vi "examen.vi"() -> ()   [LabVIEW 2020]
uses:
  <vilib>/numeric/Random Number (Range) DBL.vi
panel:
  in  "?":dbl
  in  "LIMITE MINIMO":dbl
  in  "LIMITE MAXIMO":dbl
  out "VALOR HISTERESIS":bool
  out "señal":dynamicdata(graph)
  out "?":dbl
  out "VALOR":bool
  out "señal sin filtro":dbl
  in  "?":bool
  # "EXAMEN INSTRUMENTACION VIRTUAL"
  # "Max."
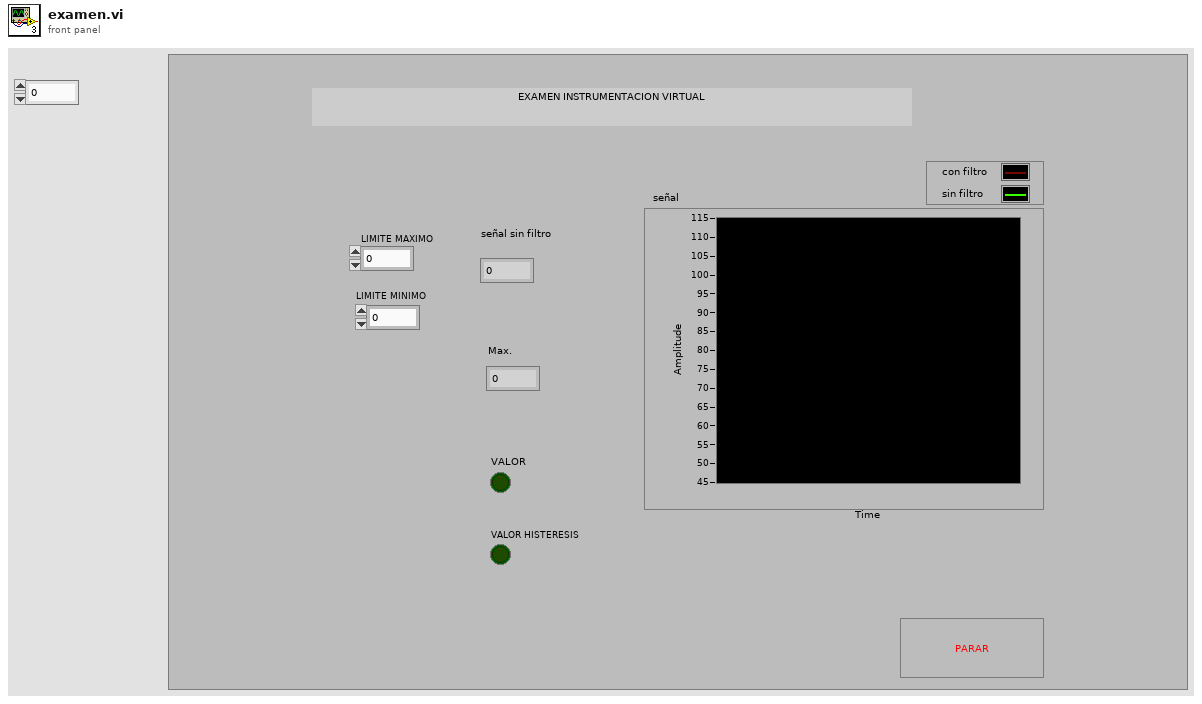
[diagram p1: front panel]
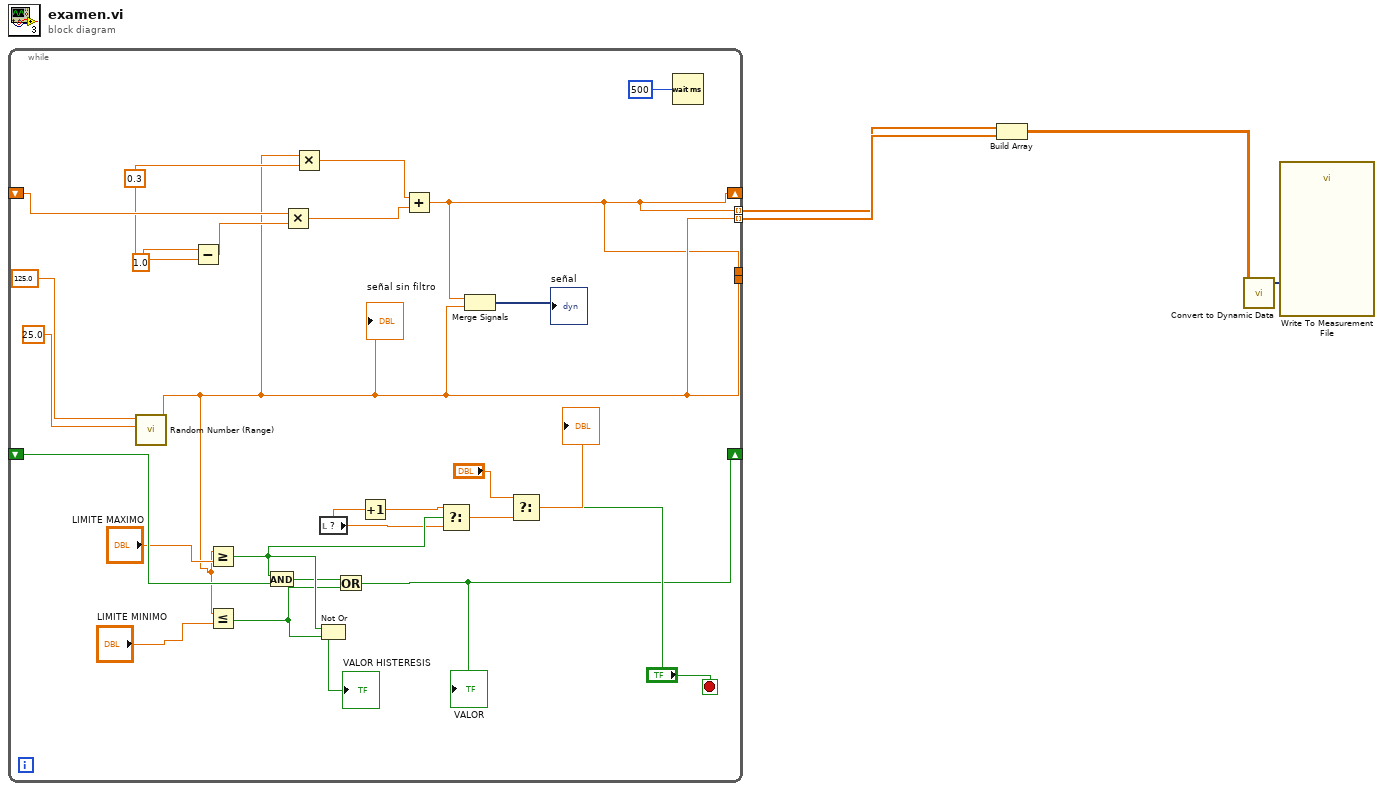
[diagram p0: block diagram]
diagram:
  n1 = while {
    shift-right: [w8] -> _
    shift-left: _ -> [w27]
    tunnel: [w9] -> _
    tunnel: [w8] -> _
    shift-right: [w7] -> _
    shift-left: _ -> [w22]
    tunnel: [w9] -> w4 mode=indexing
    tunnel: [w8] -> w3 mode=indexing
    stop <- "?" stop-if-true
    w14 = 0.3
    n2 = call-poly <vilib>:"Random Number (Range).vi"("lower bound (0)"=25.0, "upper bound (100)"=125.0) -> ("number"=w9:dbl)  [unwired: 9 in]
    "señal sin filtro" <- w9
    n3 = Subtract(x=1.0, y=w14) -> (x-y=w16:dbl)
    n4 = Greater Or Equal?(x=w9, y="LIMITE MAXIMO") -> (x >= y?=w24:bool)
    n5 = Less Or Equal?(x=w9, y="LIMITE MINIMO") -> (x <= y?=w6:bool)
    n6 = And(x=w24, y=w22) -> (x .and. y?=w23:bool)
    n7 = Multiply(x=w27, y=w16) -> (x*y=w26:dbl)
    n8 = Multiply(x=w9, y=w14) -> (x*y=w17:dbl)
    n9 = Not Or(1:w6, 2:w24) -> (0:→"VALOR HISTERESIS":bool)
    n10 = local read item#3() -> (w21:dbl)
    n11 = Or(x=w23, y=w6) -> (x .or. y?=w7:bool)
    "VALOR" <- w7
    n12 = Increment(x=w21) -> (x+1=w20:dbl)
    n13 = Add(x=w17, y=w26) -> (x+y=w8:dbl)
    n14 = Select(t=w20, s=w24, f=w21) -> (s? t:f=w25:dbl)
    n15 = Merge Signals(w8, w9) -> (→"señal":dynamicdata)
    n16 = Select(t="?", s="?", f=w25) -> (s? t:f=→"?":dbl)
    n17 = Wait (ms)(milliseconds to wait=u32 500 ("millisecond timer value")) -> ()  [unwired: 1 out]
  }
  n18 = Build Array(w3, w4) -> (w2:dbl[][])
  n19 = call "Convert to Dynamic Data"("2D Array"=w2) -> ("Dynamic Data Type"=w1:dynamicdata)  [unwired: 3 in]
  n20 = call "Write To Measurement File"("Signals"=w1) -> ()  [unwired: 16 in, 3 out]
